vi "UDP Rx.vi"(5 "max size (548)":i32=548, 7 "port":u16=60000, 8 "error in (no error)":errorcluster, 10 "Count Pointer":refnum<class "Pointer.lvclass">, 11 "Stop Pointer":refnum<class "Pointer.lvclass">) -> (0 "error out":errorcluster)   [LabVIEW 2017]
uses:
  <vilib>/NI/Memory Manager/Classes/Pointer/Pointer.lvclass
  <vilib>/NI/Memory Manager/Classes/Pointer/Pointer.lvclass/Pointer.ctl
  <vilib>/NI/Memory Manager/Classes/Pointer/Write I32.vi
  <vilib>/NI/Memory Manager/Classes/Pointer/Read Bool.vi
  <vilib>/NI/Memory Manager/Classes/Pointer/Write Bool.vi
  <vilib>/NI/Memory Manager/Classes/Pointer/Write (No Check).vi
  <vilib>/NI/Memory Manager/Classes/Pointer/Write (No Check) I32.vi
  <vilib>/NI/Memory Manager/Classes/Pointer/Check Move.vi
  <vilib>/NI/Memory Manager/Classes/Pointer/Read (No Check).vi
  <vilib>/NI/Memory Manager/Classes/Pointer/Read (No Check) Bool.vi
  <vilib>/NI/Memory Manager/Classes/Pointer/Write (No Check) Bool.vi
  <vilib>/NI/Memory Manager/Classes/Pointer/Get Address.vi
  <vilib>/NI/Memory Manager/Classes/Pointer/Check Null Pointer.vi
  <vilib>/NI/Memory Manager/Classes/Pointer/Check Count.vi
  <vilib>/NI/Memory Manager/Classes/Pointer/Check Bounds (Power of 2).vi
  <vilib>/NI/Memory Manager/Classes/Pointer/Errors.vi
  <vilib>/NI/Memory Manager/Classes/Pointer/Null Pointer.vi
  <vilib>/NI/Memory Manager/Classes/Pointer/Is Null.vi
  <vilib>/NI/Memory Manager/Classes/Pointer/Get Size.vi
  <vilib>/NI/Memory Manager/Classes/Pointer/Out of Bounds.vi
  <vilib>/NI/Memory Manager/Classes/Pointer/Check Bounds.vi
  <vilib>/NI/Memory Manager/Classes/Pointer/Create Error.vi
  <vilib>/NI/Memory Manager/VIs/Source.Write.String.vi
  <vilib>/NI/Memory Manager/Classes/Pointer/Write Pointer Size.vi
  <vilib>/NI/Memory Manager/VIs/Source.Write.Scalar.Base10.vi
  <vilib>/NI/Memory Manager/VIs/Source.Write.Scalar.Base10 (U64).vi
  <vilib>/NI/Memory Manager/Classes/Pointer/Check Pointer Bounds.vi
  <vilib>/NI/Memory Manager/Classes/Pointer/Check Buffer Bounds.vi
  <vilib>/NI/Memory Manager/VIs/New Error Cluster Constant.vi
  <vilib>/NI/Memory Manager/VIs/New Error Cluster Constant (512B).vi
  <vilib>/NI/Memory Manager/VIs/Error Cluster.Set Status.vi
  <vilib>/NI/Memory Manager/VIs/Error Cluster.Set Code.vi
  <vilib>/NI/Memory Manager/VIs/Error Cluster.Set VI Source.vi
  <vilib>/NI/Memory Manager/Constants/Constants.vi
  <vilib>/NI/Memory Manager/Constants/Library Name.vi
  <vilib>/NI/Memory Manager/Classes/Pointer/Pointer Error Info.vi
  <vilib>/NI/Memory Manager/Constants/Pointer Class Name.vi
  <vilib>/NI/Memory Manager/Classes/Pointer/Buffer Underflow.vi
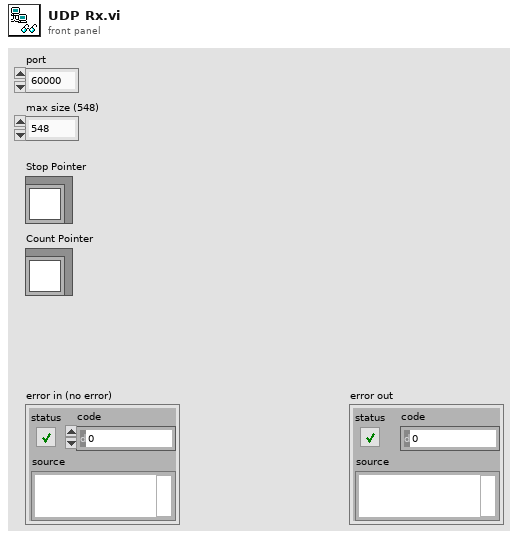
[diagram p1: front panel]
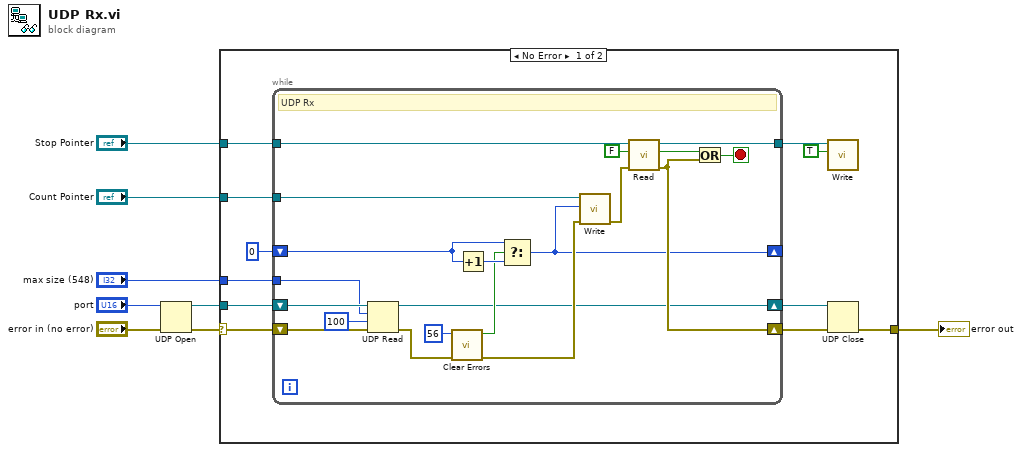
[diagram p0: block diagram]
diagram:
  n1 = UDP Open(8:"error in (no error)", 11:"port") -> (port=w8:refnum<k16>, 0:w2:errorcluster)  [unwired: 3 in, 1 out]
  n2 = case shown="No Error" w2 {
    selector: w2 -> [w12 w40]
    tunnel: w8 -> [w19 _]
    tunnel: "max size (548)" -> [w18 _]
    tunnel: "Stop Pointer" -> [w16 _]
    tunnel: "Count Pointer" -> [w15 _]
    tunnel: [w9 w40] -> w1
    frame No Error {
      n3 = while {
        shift-right: [w25] -> w11
        shift-left: w12 -> [w38]
        shift-right: [w24] -> w10
        shift-left: w19 -> [w39]
        tunnel: w16 -> [w30]
        tunnel: w18 -> [w36]
        shift-right: [w22] -> _
        shift-left: 0 -> [w32]
        tunnel: w15 -> [w28]
        tunnel: [w23] -> w14
        stop <- w37 stop-if-true
        # "UDP Rx"
        n4 = UDP Read(connection ID=w39, max size (548)=w36, timeout ms (25000)=100, 8:w38) -> (error out=w33:errorcluster, 3:w24:refnum<k16>)  [unwired: 3 out]
        n5 = call <vilib>:"Clear Errors.vi"("error in (no error)"=w33, "specific error code to clear (0: all)"=56) -> ("error out"=w27:errorcluster, "specific error cleared?"=w29:bool)  [unwired: 4 in]
        n6 = Increment(x=w32) -> (x+1=w31:i32)
        n7 = Select(t=w32, s=w29, f=w31) -> (s? t:f=w22:i32)
        n8 = call-poly <vilib>:"Write.vi"("error in (no error)"=w27, "buffer in"=w22, "Pointer in"=w28) -> ("error out"=w26:errorcluster)  [unwired: 5 in, 3 out]
        n9 = call-poly <vilib>:"Read.vi"("error in (no error)"=w26, "buffer in"=FALSE, "Pointer in"=w30) -> ("error out"=w25:errorcluster, "buffer out"=w21:bool, "Pointer out"=w23:refnum<class "Pointer.lvclass">)  [unwired: 5 in, 1 out]
        n10 = Or(x=w21, y=w25) -> (x .or. y?=w37:bool)
      }
      n11 = call-poly <vilib>:"Write.vi"("buffer in"=TRUE ("value"), "Pointer in"=w14) -> ()  [unwired: 6 in, 4 out]
      n12 = UDP Close(connection ID=w10, 8:w11) -> (error out=w9:errorcluster)  [unwired: 1 out]
    }
    frame Error {
    }
  }
  "error out" <- w1
